vi "Get Plugin Paths.vi"(8 "error in (no error)":errorcluster, 11 "MeasurementPluginService in":refnum<class "Measurement Plugin Service.lvclass">) -> (0 "error out":errorcluster, 2 "Plugin Paths":T1, 3 "MeasurementPluginService out":refnum<class "Measurement Plugin Service.lvclass">)   [LabVIEW 2020, in "MeasurementLink Measurement Server.lvlib" / "Measurement Plugin Service.lvclass"]
uses:
  Measurement Plugin Service.lvclass
  Plugin Paths.ctl
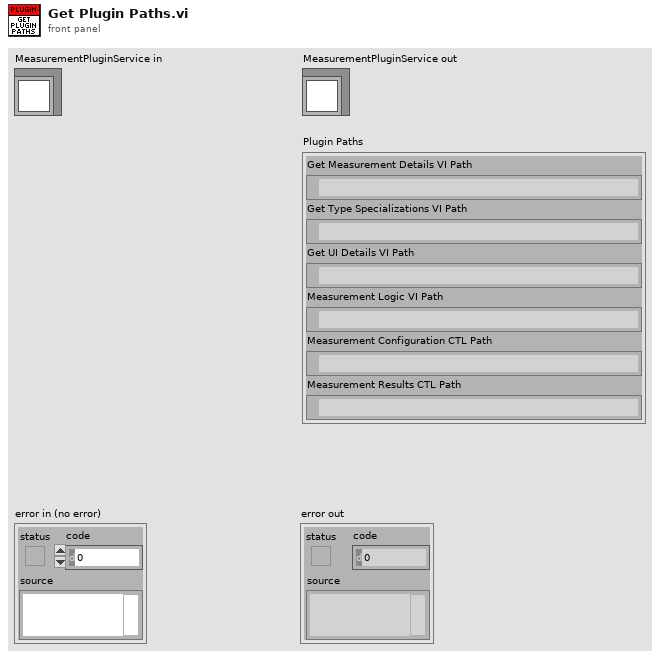
[diagram p1: front panel]
types:
  T1 = typedef "MeasurementLink Measurement Server.lvlib/Measurement Plugin Service.lvclass/Plugin Paths.ctl" = cluster{"Get Measurement Details VI Path":path, "Get Type Specializations VI Path":path, "Get UI Details VI Path":path, "Measurement Logic VI Path":path, "Measurement Configuration CTL Path":path, "Measurement Results CTL Path":path}
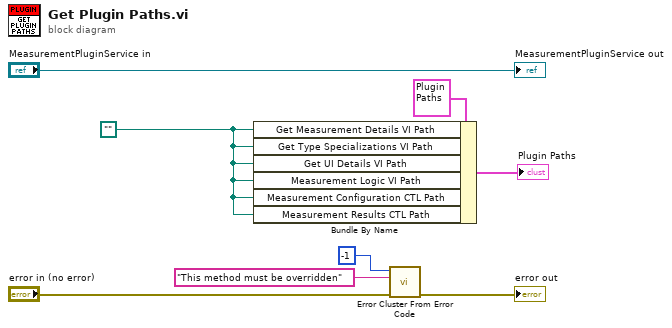
[diagram p0: block diagram]
diagram:
  w3 = path ""
  n1 = Bundle By Name(cluster=T1 {"Get Measurement Details VI Path"=path "", "Get Type Specializations VI Path"=path "", "Get UI Details VI Path"=path "", "Measurement Logic VI Path"=path "", "Measurement Configuration CTL Path"=path "", "Measurement Results CTL Path"=path ""} ("Plugin Paths"), "Get Measurement Details VI Path"=w3, "Get Type Specializations VI Path"=w3, "Get UI Details VI Path"=w3, "Measurement Logic VI Path"=w3, "Measurement Configuration CTL Path"=w3, "Measurement Results CTL Path"=w3) -> (→"Plugin Paths":T1)
  n2 = call <vilib>:"Error Cluster From Error Code.vi"("error in (no error)"="error in (no error)", "error message (\"\")"="This method must be overridden" ("error message (\"\")"), "error code (0)"=-1) -> ("error out"=→"error out":errorcluster)  [unwired: 6 in]
  "MeasurementPluginService out" <- "MeasurementPluginService in"
